vi "Read Page Menu Properties.vi"(8 "Error In":errorcluster, 11 "Custom Device Page .NET Ref In":refnum<k24>) -> (0 "Error Out":errorcluster, 2 "All Menu Properties":T1[](array[typedef]), 3 "Custom Device Page .NET Ref Out":refnum<k24>)   [LabVIEW 2015, in "VeriStand XML Parser.lvlib"]
doc: "Reads and returns the properties of all menus of the page"
uses:
  VeriStand XML Parser.lvlib
  XML Controls/RuntTimeMenu Properties.ctl
  XML Controls/Execution Types.ctl
  XML Controls/Path Cluster.ctl
  XML Controls/Dependency Properties.ctl
  NationalInstruments.VeriStand.XMLReader
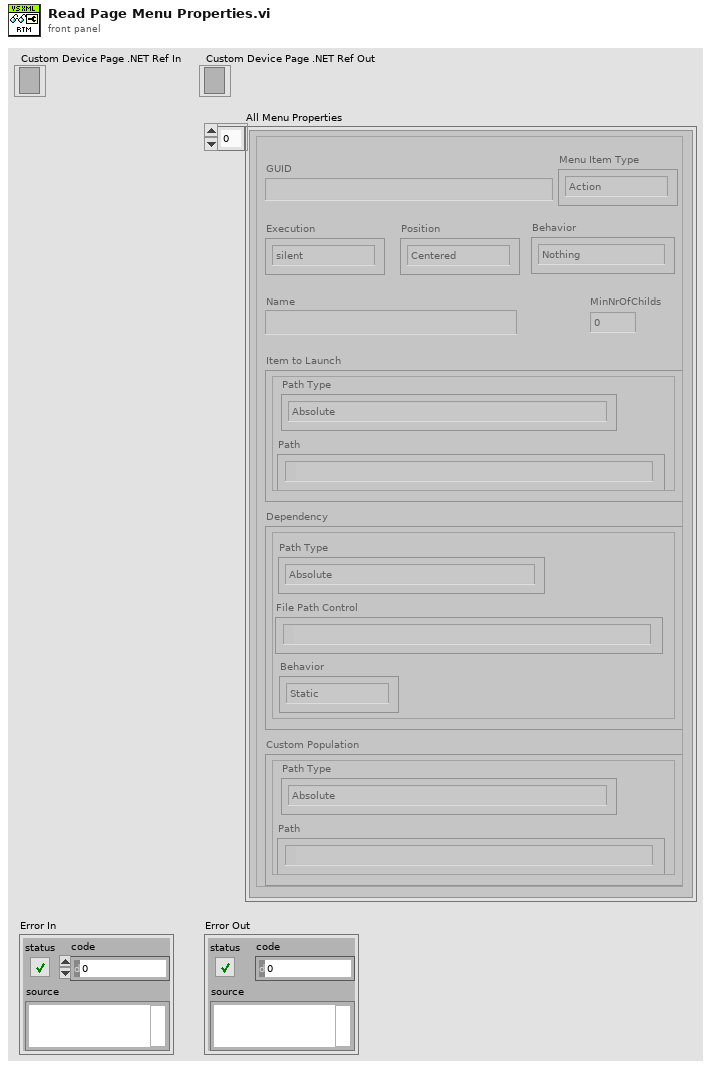
[diagram p1: front panel]
types:
  T1 = typedef "VeriStand XML Parser.lvlib/RuntTimeMenu Properties.ctl" = cluster{"GUID":string, "Execution":T2, "MinNrOfChilds":u32, "Name":string, "Item to Launch":T3, "Dependency":T4, "Custom Population":T3, "Menu Item Type":enum16{"Action", "VI", "Separator", "Custom"}, "Behavior":enum16{"Nothing", "Open Front Panel"}, "Position":enum16{"Centered", "Mouse Pointer"}}
  T2 = typedef "VeriStand XML Parser.lvlib/Execution Types.ctl" = enum16{"silent", "modal", "floating", "default"}
  T3 = typedef "VeriStand XML Parser.lvlib/Path Cluster.ctl" = cluster{"Path":path, "Path Type":enum16{"Absolute", "To Base", "To Common Doc Dir", "To Application Data Dir"}}
  T4 = typedef "VeriStand XML Parser.lvlib/Dependency Properties.ctl" = cluster{"File Path Control":path, "Path Type":enum16{"Absolute", "To Base", "To Common Doc Dir", "To Application Data Dir"}, "Behavior":enum16{"Static", "Dynamic"}}
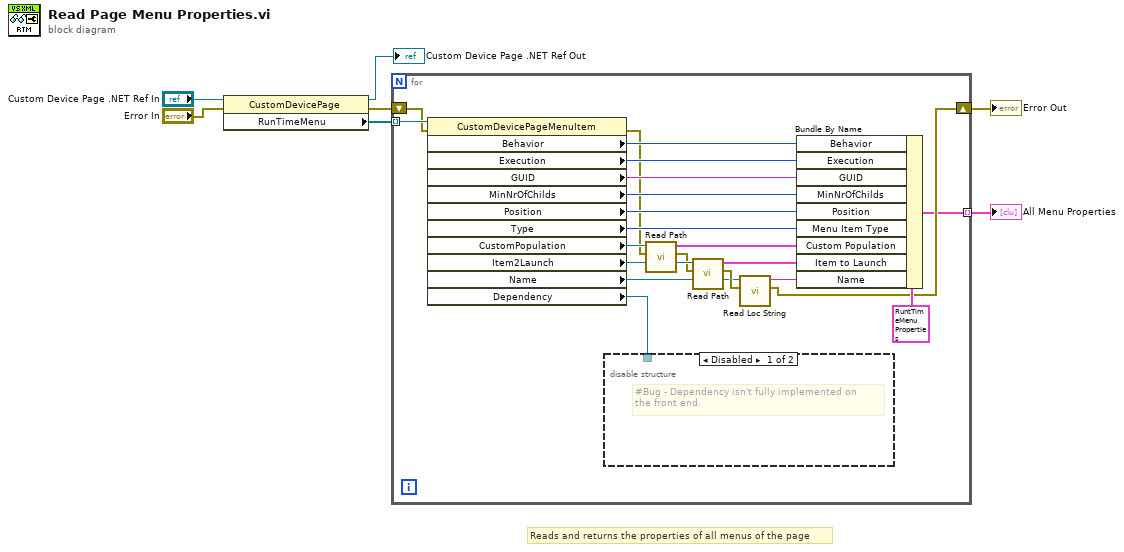
[diagram p0: block diagram]
diagram:
  # "Reads and returns the properties of all menus of the page"
  n1 = property class="CustomDevicePage"(reference="Custom Device Page .NET Ref In", error in="Error In") -> (reference out=→"Custom Device Page .NET Ref Out":refnum<k24>, error out=w4:errorcluster, "RunTimeMenu"=w3:refnum<k24>[])
  n2 = for {
    tunnel: w3 -> [w27] mode=indexing
    shift-right: [w9] -> w7
    shift-left: w4 -> [w26]
    tunnel: [w8] -> w6 mode=indexing
    n3 = property class="CustomDevicePageMenuItem"(reference=w27, error in=w26) -> (error out=w18:errorcluster, "Behavior"=w25:i32, "Execution"=w24:i32, "GUID"=w23:string, "MinNrOfChilds"=w22:i32, "Position"=w21:i32, "Type"=w20:i32, "CustomPopulation"=w19:refnum<k24>, "Item2Launch"=w17:refnum<k24>, "Name"=w12:refnum<k24>, "Dependency"=w10:refnum<k24>)  [unwired: 1 out]
    n4 = disable-structure shown="Disabled" {
      disable-tunnel: w10 -> [_ _]
      frame Disabled {
        # "#Bug - Dependency isn't fully implemented on\nthe front end."
      }
      frame Enabled {
      }
    }
    n5 = call "Read Path.vi"("Error In"=w18, "Path .NET Ref"=w19) -> ("Error Out"=w16:errorcluster, "Path Properties"=w15:T3)  [unwired: 8 in]
    n6 = call "Read Path.vi"("Error In"=w16, "Path .NET Ref"=w17) -> ("Error Out"=w13:errorcluster, "Path Properties"=w14:T3)  [unwired: 8 in]
    n7 = call "Read Loc String.vi"("Error In"=w13, "Loc String .NET Ref"=w12) -> ("Error Out"=w9:errorcluster, "English"=w11:string)  [unwired: 7 in, 1 out]
    n8 = Bundle By Name(cluster=T1 {"GUID"="", "Execution"=enum."silent", "MinNrOfChilds"=0, "Name"="", "Item to Launch"={"Path"=path "", "Path Type"=enum."Absolute"}, "Dependency"={"File Path Control"=path "", "Path Type"=enum."Absolute", "Behavior"=enum."Static"}, "Custom Population"={"Path"=path "", "Path Type"=enum."Absolute"}, "Menu Item Type"=enum."Action", "Behavior"=enum."Nothing", "Position"=enum."Centered"} ("Menu Item"), "Behavior"=w25, "Execution"=w24, "GUID"=w23, "MinNrOfChilds"=w22, "Position"=w21, "Menu Item Type"=w20, "Custom Population"=w15, "Item to Launch"=w14, "Name"=w11) -> (w8:T1)
  }
  "Error Out" <- w7
  "All Menu Properties" <- w6
